vi "Calculate frames and dt.vi"() -> (1 "Period":i32, 2 "# slices/frames":i32, 4 "PI MVR(inc)":string, 5 "# stacks":i32, 6 "Start - inc":dbl)   [LabVIEW 2020]
uses:
  _Globals/Global Controls.vi
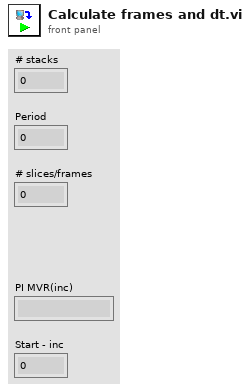
[diagram p1: front panel]
types:
  T1 = typedef "Exp Params.ctl" = cluster{"Experiment Type":string, "Experiment Name":string, "ExpPath":path, "TSFrames":i32, "TSfps":i32, "ZTSFrames":i32, "ZTSdt":i32, "Streaming":bool, "Z Stack Settings":cluster{"Start":dbl, "Step Size":dbl, "Finish":dbl}, "total images":i32, "tdms ref":refnum<k34>, "frame #":i64, "images per stack":i32, "total stacks":i32, "period":i32, "PI command":string}
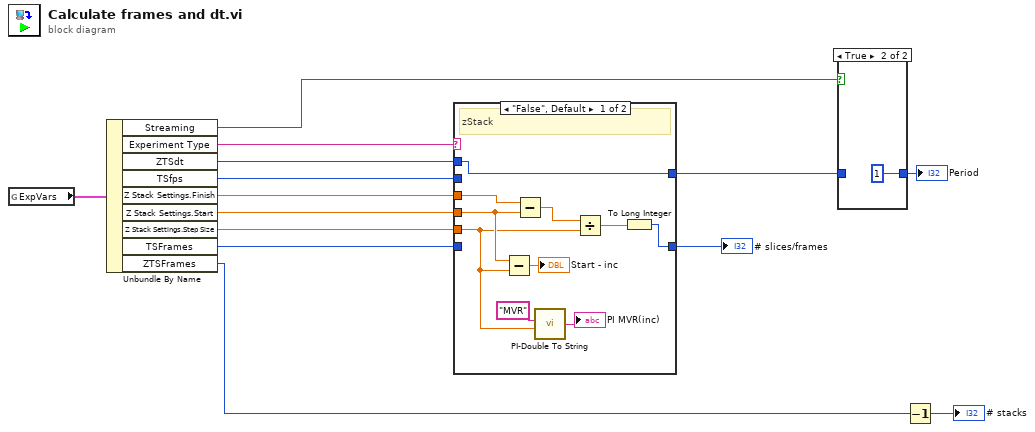
[diagram p0: block diagram]
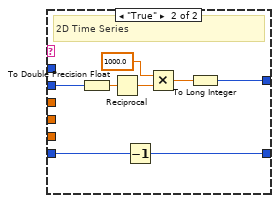
[diagram p3: hidden frame]
diagram:
  n1 = global read "Global Controls.vi" "ExpVars"() -> (w3:T1)
  n2 = Unbundle By Name(w3) -> ("Streaming"=w11:bool, "Experiment Type"=w1:string, "ZTSdt"=w13:i32, "TSfps"=w12:i32, "Z Stack Settings.Finish"=w8:dbl, "Z Stack Settings.Start"=w7:dbl, "Z Stack Settings.Step Size"=w6:dbl, "TSFrames"=w5:i32, "ZTSFrames"=w2:i32)
  n3 = case shown="\"False\", Default" w1 {
    tunnel: w13 -> [w24 _]
    tunnel: w12 -> [_ w27]
    tunnel: [w24 w30] -> w10
    tunnel: w8 -> [w20 _]
    tunnel: w7 -> [w17 _]
    tunnel: w6 -> [w16 _]
    tunnel: [w18 w28] -> w4
    tunnel: w5 -> [_ w29]
    frame "False", Default {
      # "zStack"
      n4 = Subtract(x=w17, y=w16) -> (x-y=→"Start - inc":dbl)
      n5 = Subtract(x=w20, y=w17) -> (x-y=w23:dbl)
      n6 = call "PI-Double To String.vi"("Start"=w16, "String in"="MVR") -> ("String out"=→"PI MVR(inc)":string)  [unwired: 2 in]
      n7 = Divide(x=w23, y=w16) -> (x/y=w19:dbl)
      n8 = To Long Integer(number=w19) -> (32bit integer=w18:i32)
    }
    frame "True" {
      # "2D Time Series"
      n9 = To Double Precision Float(number=w27) -> (double precision float=w25:dbl)
      n10 = Reciprocal(x=w25) -> (1/x=w31:dbl)
      n11 = Decrement(x=w29) -> (x-1=w28:i32)
      n12 = Multiply(x=1000.0 ("y"), y=w31) -> (x*y=w32:dbl)
      n13 = To Long Integer(number=w32) -> (32bit integer=w30:i32)
    }
  }
  "# slices/frames" <- w4
  n14 = case shown="True" w11 {
    tunnel: [w33 1 ("Period")] -> w9
    tunnel: w10 -> [w33 _]
    frame False {
    }
    frame True {
    }
  }
  "Period" <- w9
  n15 = Decrement(x=w2) -> (x-1=→"# stacks":i32)
